vi "LEBITplc.CreateSpecialDBArrays.vi"(2 "DBArray":string[][](array[string])) -> (15 "CondSpecialArray":string[][](array[string]), 16 "CondSpecialIndex":i32[](array[numeric]), 17 "CondSpecialMonValue":dbl[](array[numeric]), 18 "Dependent Monitors":string[][](array[string]))   [LabVIEW 2014, in "LEBITplc.lvlib"]
uses:
  LEBITplc.lvlib
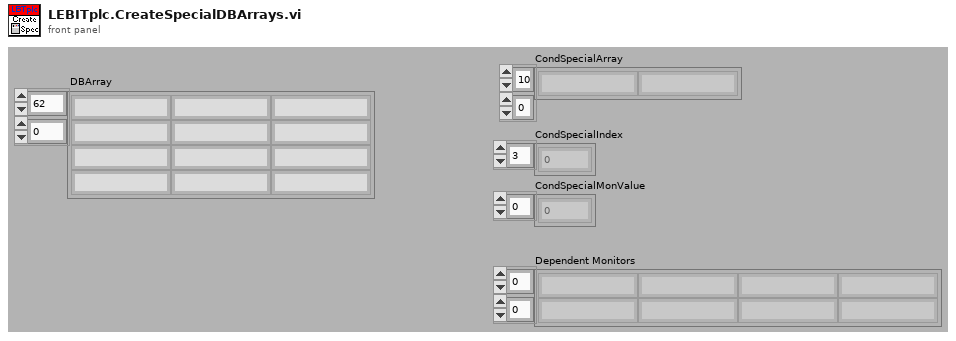
[diagram p1: front panel]
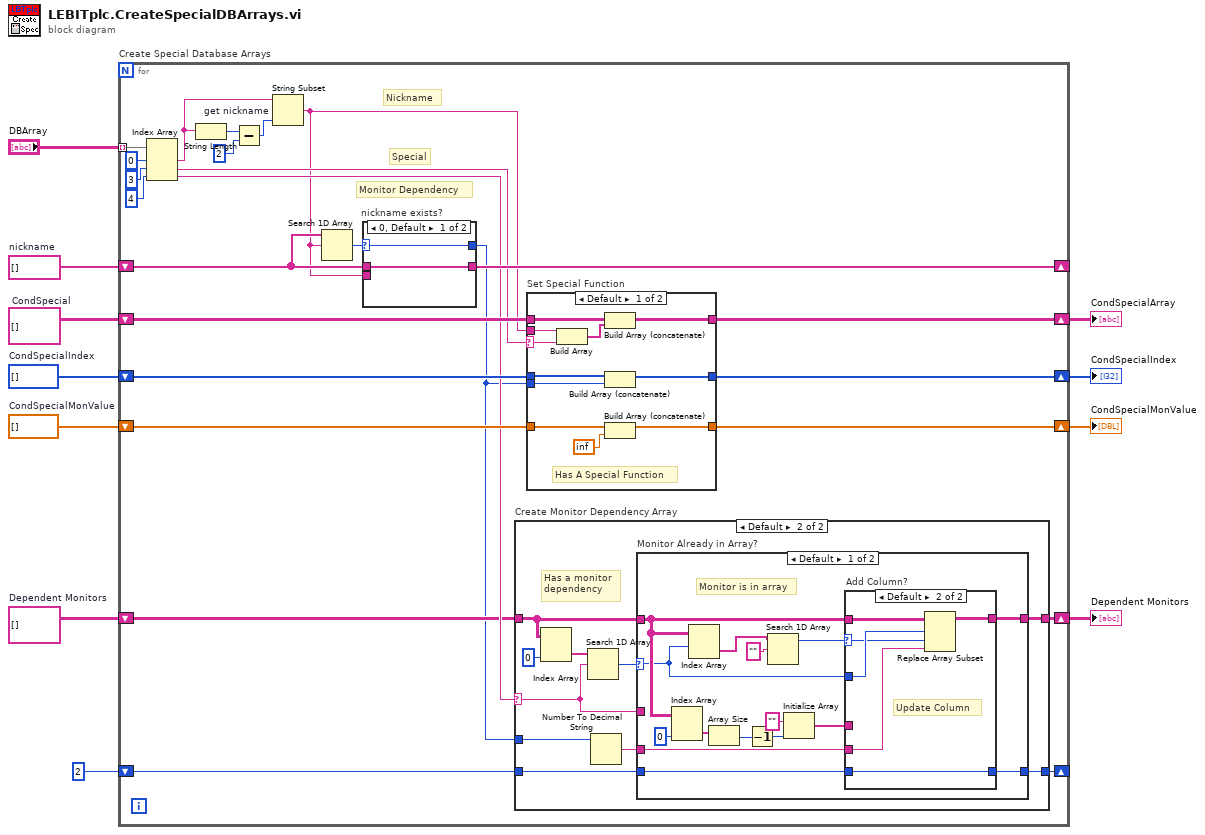
[diagram p0: block diagram]
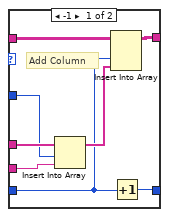
[diagram p3: hidden frame]
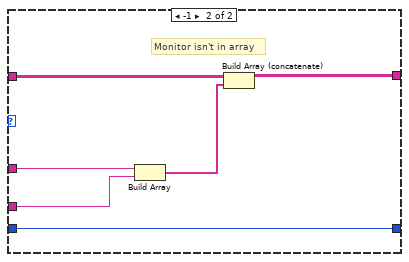
[diagram p4: hidden frame]
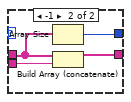
[diagram p6: hidden frame]
diagram:
  w4 = string[][] []  # Dependent Monitors
  w6 = dbl[] []  # CondSpecialMonValue
  w9 = i32[] []  # CondSpecialIndex
  w10 = string[][] []  # CondSpecial
  w11 = string[] []  # nickname
  n1 = for "Create Special Database Arrays" {
    tunnel: "DBArray" -> [w36] mode=indexing
    shift-right: [w28] -> _
    shift-left: w11 -> [w29]
    shift-right: [w27] -> w8
    shift-left: w10 -> [w24]
    shift-right: [w26] -> w7
    shift-left: w9 -> [w23]
    shift-right: [w25] -> w5
    shift-left: w6 -> [w22]
    shift-right: [w15] -> w3
    shift-left: w4 -> [w17]
    shift-right: [w12] -> _
    shift-left: 2 -> [w13]
    # "Monitor Dependency"
    # "Nickname"
    # "Special"
    n2 = Index Array(array=w36, index #1=0 ("index"), index #2=3 ("index"), index #3=4 ("index")) -> (element #1=w32:string, element #2=w19:string, element #3=w18:string)
    n3 = String Length(string=w32) -> (length=w34:i32)
    n4 = Subtract(x=w34, y=2) -> (x-y=w31:i32)
    n5 = String Subset "get nickname"(string=w32, length (rest)=w31) -> (substring=w14:string)  [unwired: 1 in]
    n6 = Search 1D Array(1D array=w29, element=w14) -> (index of element=w30:i32)  [unwired: 1 in]
    n7 = case "nickname exists?" shown="0, Default" w30 {
      selector: w30 -> [w98 _]
      tunnel: w29 -> [w99 w101]
      tunnel: w14 -> [_ w100]
      tunnel: [w99 w102] -> w28
      tunnel: [w98 w103] -> w16
      frame 0, Default {
      }
      frame -1 {
        n8 = Array Size(array=w101) -> (size(s)=w103:i32)
        n9 = Build Array (concatenate)(w101, w100) -> (w102:string[])
      }
    }
    n10 = case "Create Monitor Dependency Array" shown="Default" w18 {
      selector: w18 -> [_ w42]
      tunnel: w17 -> [w38 w47]
      tunnel: w16 -> [_ w45]
      tunnel: [w38 w46] -> w15
      tunnel: w13 -> [w37 w40]
      tunnel: [w37 w39] -> w12
      frame "" {
        # "Doesn't have a monitor dependency"
      }
      frame Default {
        # "Has a monitor\ndependency"
        n11 = Index Array(array=w47, index (col)=0 ("disabled index (col)")) -> (element=w48:string[])  [unwired: 1 in]
        n12 = Search 1D Array(1D array=w48, element=w42) -> (index of element=w43:i32)  [unwired: 1 in]
        n13 = Number To Decimal String(number=w45) -> (decimal integer string=w44:string)  [unwired: 1 in]
        n14 = case "Monitor Already in Array?" shown="Default" w43 {
          selector: w43 -> [w58 _]
          tunnel: w47 -> [w63 w80]
          tunnel: [w57 w83] -> w46
          tunnel: w44 -> [w60 w78]
          tunnel: w42 -> [_ w81]
          tunnel: w40 -> [w55 w79]
          tunnel: [w56 w79] -> w39
          frame Default {
            # "Monitor is in array"
            n15 = Index Array(array=w63, index (col)=0 ("disabled index (col)")) -> (element=w62:string[])  [unwired: 1 in]
            n16 = Index Array(array=w63, index (row)=w58) -> (element=w50:string[])  [unwired: 1 in]
            n17 = Array Size(array=w62) -> (size(s)=w54:i32)
            n18 = Decrement(x=w54) -> (x-1=w53:i32)
            n19 = Search 1D Array(1D array=w50, element="") -> (index of element=w51:i32)  [unwired: 1 in]
            n20 = Initialize Array("", w53) -> (w49:string[])
            n21 = case "Add Column?" shown="Default" w51 {
              selector: w51 -> [_ w72]
              tunnel: w63 -> [w68 w77]
              tunnel: w58 -> [w70 w74]
              tunnel: w60 -> [w69 w73]
              tunnel: w49 -> [w71 _]
              tunnel: [w66 w76] -> w57
              tunnel: w55 -> [w64 w75]
              tunnel: [w65 w75] -> w56
              frame -1 {
                # "Add Column"
                n22 = Insert Into Array(array=w71, index=w70, new element=w69) -> (w67:string[])
                n23 = Insert Into Array(array=w68, index (col)=w64, new element=w67) -> (w66:string[][])  [unwired: 1 in]
                n24 = Increment(x=w64) -> (x+1=w65:i32)
              }
              frame Default {
                # "Update Column"
                n25 = Replace Array Subset(array=w77, new element=w73, index (row)=w74, index (col)=w72) -> (w76:string[][])
              }
            }
          }
          frame -1 {
            # "Monitor isn't in array"
            n26 = Build Array(w81, w78) -> (w82:string[])
            n27 = Build Array (concatenate)(w80, w82) -> (w83:string[][])
          }
        }
      }
    }
    n28 = case "Set Special Function" shown="Default" w19 {
      selector: w19 -> [w90 _]
      tunnel: w24 -> [w94 w97]
      tunnel: [w93 w97] -> w27
      tunnel: w14 -> [w91 _]
      tunnel: w23 -> [w89 w96]
      tunnel: [w88 w96] -> w26
      tunnel: w16 -> [w87 _]
      tunnel: w22 -> [w86 w95]
      tunnel: [w85 w95] -> w25
      frame Default {
        # "Has A Special Function"
        n29 = Build Array(w91, w90) -> (w92:string[])
        n30 = Build Array (concatenate)(w94, w92) -> (w93:string[][])
        n31 = Build Array (concatenate)(w89, w87) -> (w88:i32[])
        n32 = Build Array (concatenate)(w86, inf) -> (w85:dbl[])
      }
      frame "" {
        # "Doesn't have A Special Function"
      }
    }
  }
  "CondSpecialArray" <- w8
  "CondSpecialIndex" <- w7
  "CondSpecialMonValue" <- w5
  "Dependent Monitors" <- w3
